vi "Create Queue.vi"(9 "Queue jettl":refnum<class "Queue.lvclass">, 10 "Alias":string, 11 "Hello World Queue in":refnum<class "Hello World Queue.lvclass">) -> (3 "Hello World Queue out":refnum<class "Hello World Queue.lvclass">)   [LabVIEW 2021, in "Hello World Queue.lvlib" / "Hello World Queue.lvclass"]
uses:
  Hello World Queue.lvclass
  jettl/Queue/Queue.lvclass
  Hello World Queue.lvclass/Hello World Queue.ctl
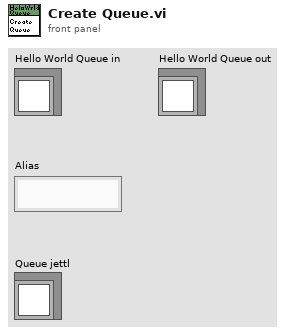
[diagram p1: front panel]
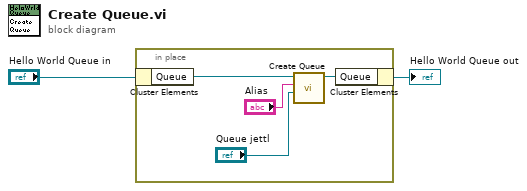
[diagram p0: block diagram]
diagram:
  n1 = in-place {
    n2 = in-place-cluster #1("Hello World Queue in") -> ("Queue"=w4:refnum<class "Queue.lvclass">)
    n3 = call-dynamic "Create Queue.vi"("Queue"="Queue jettl", "Self Queue Alias"="Alias", "Create Queue in"=w4) -> ("Create Queue out"=w3:refnum<class "Queue.lvclass">)  [unwired: 8 in]
    n4 = in-place-cluster #1("Queue"=w3) -> (→"Hello World Queue out":refnum<class "Hello World Queue.lvclass">)
  }
